vi "Label Targets AprilTagl.vi"(9 "results":T1={"diameter points"={"first point"={"x"=0.0, "y"=0.0}, "projected point"={"x"=0.0, "y"=0.0}}, "Tag Center"={"X"=0.0, "Y"=0.0}, "AprilTag #"=68, "homography matrix"=[], "corner points"=[]} {"Tag Center"."Y" format="%0.2f"; "Tag Center"."X" format="%0.2f"}, 11 "Image in":T2) -> (3 "Image out":T2)   [LabVIEW 2025]
doc: "Draw scores near or on the particle and an ellipse around the target. Scores that are below the score threshold are drawn in red, above in green."
uses:
  <vilib>/vision/Image Controls.llb/IMAQ Image.ctl
  AprilTag Target Fields.ctl
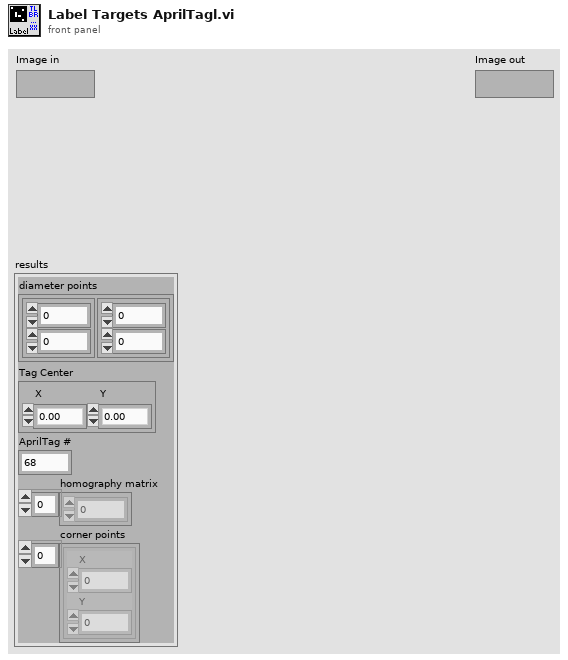
[diagram p1: front panel]
types:
  T1 = typedef "AprilTag Target Fields.ctl" = cluster{"diameter points":cluster{"first point":cluster{"x":dbl, "y":dbl}, "projected point":cluster{"x":dbl, "y":dbl}}, "Tag Center":cluster{"X":dbl, "Y":dbl}, "AprilTag #":i32, "homography matrix":dbl[], "corner points":cluster{"X":dbl, "Y":dbl}[]}
  T2 = typedef "IMAQ Image.ctl" = refnum<image>
  T3 = cluster{"Desired Font (Application)":enum16{"User-specified Font", "Application Font", "System Font", "Dialog Font"}, "[User-specified Font]":cluster{"Font Name":string, "Size":i16, "Strikeout?":bool, "Italic?":bool, "Underline?":bool, "Outline?":bool, "Shadow?":bool, "Bold?":bool, "Rotation Angle":dbl}, "Horizontal Alignment":i16, "Vertical Alignment":i16}
  T4 = cluster{"first point":cluster{"x":dbl, "y":dbl}, "projected point":cluster{"x":dbl, "y":dbl}}
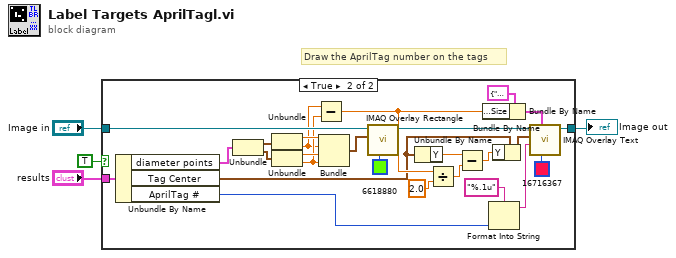
[diagram p0: block diagram]
diagram:
  # "Draw the AprilTag number on the tags"
  n1 = case shown="True" TRUE {
    tunnel: [w5 w31] -> w4
    tunnel: "Image in" -> [w5 w30]
    tunnel: "results" -> [_ w29]
    frame False {
    }
    frame True {
      n2 = Unbundle By Name(w29) -> ("diameter points"=w27:T4, "Tag Center"=w6:cluster{"X":dbl, "Y":dbl}, "AprilTag #"=w7:i32)
      n3 = Unbundle(w27) -> ("first point"=w14:cluster{"x":dbl, "y":dbl}, "projected point"=w19:cluster{"x":dbl, "y":dbl})
      n4 = Unbundle(w14) -> ("x"=w26:dbl, "y"=w15:dbl)
      n5 = Unbundle(w19) -> ("x"=w25:dbl, "y"=w17:dbl)
      n6 = Subtract(x=w15, y=w17) -> (x-y=w8:dbl)
      n7 = Bundle("x"=w26, "y"=w15, "x"=w25, "y"=w17) -> (w24:cluster{"x":dbl, "y":dbl, "x":dbl, "y":dbl})  [unwired: 1 in]
      n8 = call "IMAQ Overlay Rectangle"("Color"=u32 6618880, "Rectangle"=w24, "Image"=w30) -> ("Image Out"=w16:T2)  [unwired: 7 in, 1 out]
      n9 = Unbundle By Name(w6) -> ("Y"=w12:dbl)
      n10 = Divide(x=w8, y=2.0) -> (x/y=w9:dbl)
      n11 = Subtract(x=w12, y=w9) -> (x-y=w11:dbl)
      n12 = Bundle By Name(cluster=T3 {"Desired Font (Application)"=enum."User-specified Font", "[User-specified Font]"={"Font Name"="Ariel", "Size"=25, "Strikeout?"=FALSE, "Italic?"=FALSE, "Underline?"=FALSE, "Outline?"=FALSE, "Shadow?"=TRUE, "Bold?"=TRUE, "Rotation Angle"=0.0}, "Horizontal Alignment"=1, "Vertical Alignment"=1} ("Font, Size & Style"), "[User-specified Font].Size"=w8) -> (w18:T3)
      n13 = Format Into String(format string="%.1u", w7) -> (resulting string=w21:string)  [unwired: 2 in, 1 out]
      n14 = Bundle By Name(cluster=w6, "Y"=w11) -> (w13:cluster{"X":dbl, "Y":dbl})
      n15 = call "IMAQ Overlay Text"("Text Color (black)"=u32 16716367 ("Color"), "Font, Size & Style"=w18, "String"=w21, "Origin"=w13, "Image"=w16) -> ("Image Out"=w31:T2)  [unwired: 5 in, 1 out]
    }
  }
  "Image out" <- w4
